vi "flattenMassToXML.vi"   [LabVIEW 2012, in "UnitsAndXML.lvlib"]
doc: "Generates an XML string for <B>mass</B> in the unit specified in <B>massUnitInXML</B>. Connect <B>mass</B> and <B>massAgain</B> to the same source. The VI uses <B>massAgain</B> to obtain the data name."
uses:
  <userlib>/Common/UnitsAndXML/UnitsAndXML.lvlib
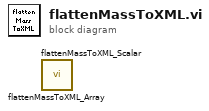
[diagram p0: block diagram]
diagram:
  n1 = call <userlib>:"flattenMassToXML_Array.vi"() -> ()  [unwired: 10 in, 2 out]
  n2 = call <userlib>:"flattenMassToXML_Scalar.vi"() -> ()  [unwired: 10 in, 2 out]
